vi "Write ModelValidationConfig.vi"(8 "error in (no error)":errorcluster, 10 "ModelValidationConfig":T1={"NoiseVariance"=0.001, "Iindex"=3, "OffsetTime"=2.0, "InterpolationFactor"=3, "Initial condition"={"H0"=4.55, "xd0"=0.275, "D0"=4.2}}, 11 "ModelValidationPlugin in":refnum<class "ModelValidationPlugin.lvclass">) -> (0 "error out":errorcluster, 3 "ModelValidationPlugin out":refnum<class "ModelValidationPlugin.lvclass">)   [LabVIEW 2017, in "AppPlugins.lvlib" / "ModelValidationPlugin.lvclass"]
uses:
  ModelValidationPlugin.lvclass
  PublicAPI/TypeDef/Config.ctl
  ModelValidationPlugin.lvclass/ModelValidationPlugin.ctl
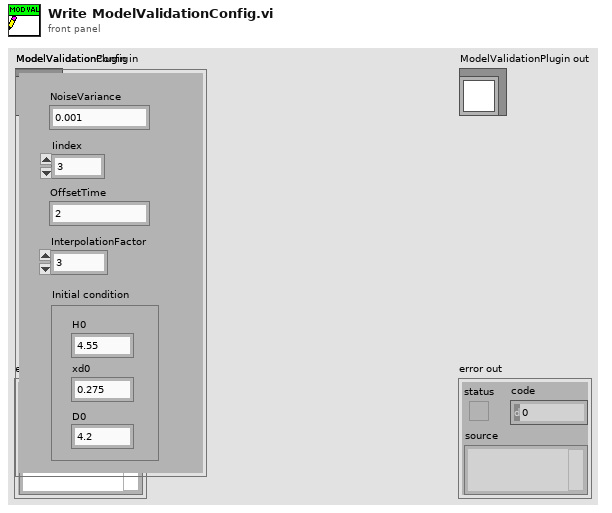
[diagram p1: front panel]
types:
  T1 = typedef "AppPlugins.lvlib/ModelValidationPlugin.lvclass/Config.ctl" = cluster{"NoiseVariance":dbl, "Iindex":i32, "OffsetTime":dbl, "InterpolationFactor":i32, "Initial condition":cluster{"H0":dbl, "xd0":dbl, "D0":dbl}}
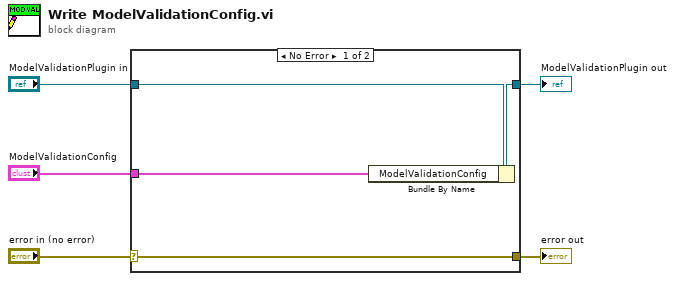
[diagram p0: block diagram]
diagram:
  n1 = case shown="No Error" "error in (no error)" {
    selector: "error in (no error)" -> [w9 w10]
    tunnel: [w9 w10] -> w4
    tunnel: [w7 w11] -> w2
    tunnel: "ModelValidationPlugin in" -> [w8 w11]
    tunnel: "ModelValidationConfig" -> [w6 _]
    frame No Error {
      n2 = Bundle By Name(cluster=w8, "ModelValidationConfig"=w6) -> (w7:refnum<class "ModelValidationPlugin.lvclass">)
    }
    frame Error {
    }
  }
  "error out" <- w4
  "ModelValidationPlugin out" <- w2
